vi "onTestSlippage.vi"(7 "Project in":refnum<class "TraceabilityMatrix.lvclass">, 11 "Leaf.TestCase":refnum<class "Leaf.TestCase.lvclass">) -> (0 "error out":errorcluster, 3 "Leaf.TestCase":refnum<class "Leaf.TestCase.lvclass">)   [LabVIEW 2021, in "Bananas.lvlib" / "TraceabilityMatrix.lvclass"]
uses:
  TraceabilityMatrix.lvclass
  Leaf.TestCase/Leaf.TestCase.lvclass
  C:/Repositories/LVOS/Bananas/lv-src/Bananas/Leaf/Leaf.lvclass
  TraceabilityMatrix.lvclass/TraceabilityMatrix.ctl
  Leaf/Leaf.lvclass
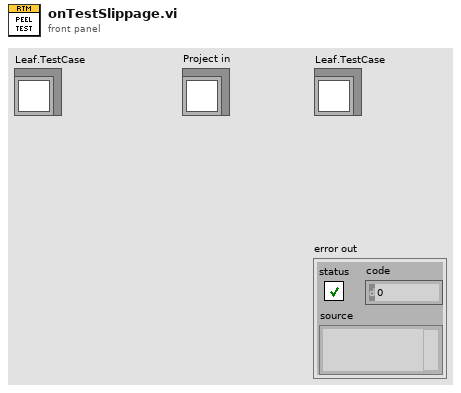
[diagram p1: front panel]
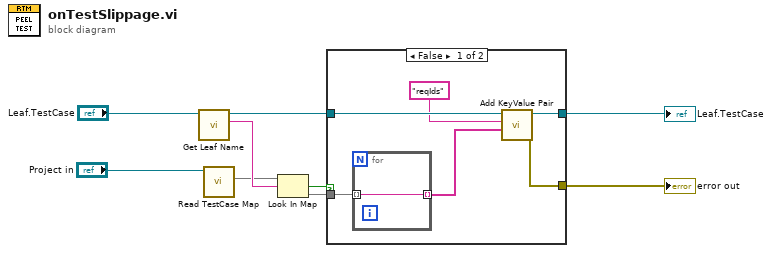
[diagram p0: block diagram]
diagram:
  n1 = call "Get Leaf Name.vi"("Leaf in"="Leaf.TestCase") -> ("Name"=w7:string, "Leaf out"=w6:refnum<class "Leaf.TestCase.lvclass">)  [unwired: 8 in, 1 out]
  n2 = call "Read TestCase Map.vi"("TraceabilityMatrix in"="Project in") -> ("TestCaseMap"=w5:map{string, set{string}})  [unwired: 9 in, 1 out]
  n3 = Look In Map(map=w5, key=w7) -> (key not found?=w9:bool, value=w8:set{string})  [unwired: 1 in]
  n4 = case shown="False" w9 {
    tunnel: [w13 w17] -> w2
    tunnel: w6 -> [w15 w17]
    tunnel: w8 -> [w11 _]
    tunnel: [w12 _] -> w1
    frame False {
      n5 = for {
        tunnel: w11 -> [w16] mode=indexing
        tunnel: [w16] -> w10 mode=indexing
      }
      n6 = call "Add KeyValue Pair.vi"("value"=w10, "key"="reqIds", "Leaf in"=w15) -> ("error out"=w12:errorcluster, "Leaf out"=w13:refnum<class "Leaf.TestCase.lvclass">)  [unwired: 7 in]
    }
    frame True {
    }
  }
  "error out" <- w1
  "Leaf.TestCase" <- w2
